vi "Select Dialog From Action.vi"(11 "Action":T2=enum."Terminal Properties") -> (3 "Dialog Selection":T1(ring))   [LabVIEW 2023]
uses:
  controls/action enum.ctl
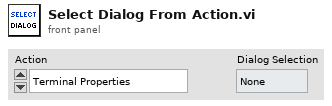
[diagram p1: front panel]
types:
  T1 = enum16{"None", "Cluster", "Property", "Method", "Class"}
  T2 = typedef "action enum.ctl" = enum16{"[NONE]", "Wire Bundle", "Wire Unbundle", "Terminal Unbundle", "Terminal Bundle", "Bundler Move Up", "Bundler Move Down", "Bundler Insert", "Bundler Remove", "Bundler Remove Unwired", "Bundler Rearrange", "In Place Insert", "In Place Remove", "In Place Remove Unwired", "In Place Rearrange", "Wire Properties", "Wire Method", "Terminal Properties", "Terminal Method", "Property Move Up", "Property Move Down", "Properties Insert", "Properties Remove", "Properties Remove Unwired", "Properties Rearrange", "Method Change", "Class for Constant", "Class For Control", "Class For Node", "Class Name to Clipboard"}
  T3 = cluster{"Action":T2, "Dialog Selection":enum16{"None", "Cluster", "Property", "Method", "Class"}}[]
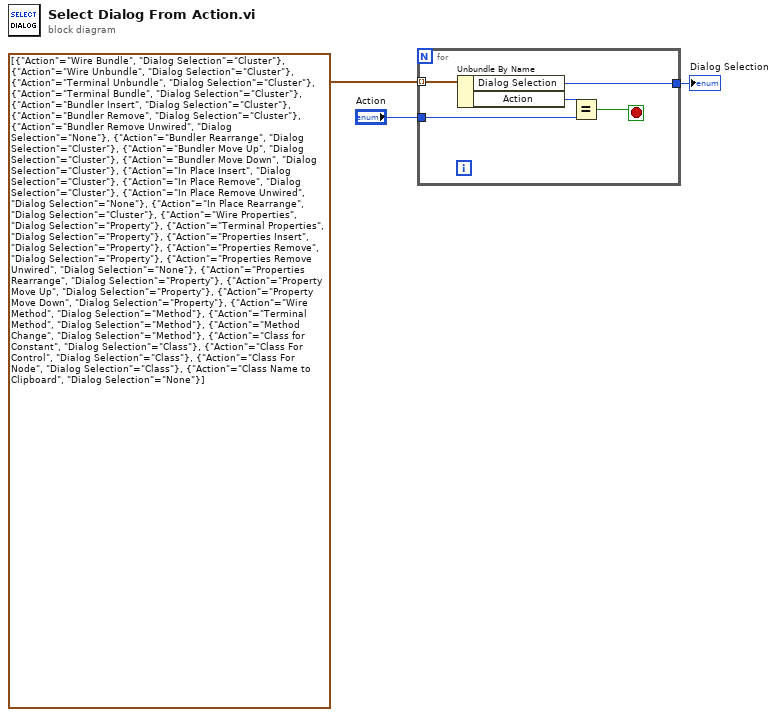
[diagram p0: block diagram]
diagram:
  n1 = for {
    tunnel: T3 [{"Action"=enum."Wire Bundle", "Dialog Selection"=enum."Cluster"}, {"Action"=enum."Wire Unbundle", "Dialog Selection"=enum."Cluster"}, {"Action"=enum."Terminal Unbundle", "Dialog Selection"=enum."Cluster"}, {"Action"=enum."Terminal Bundle", "Dialog Selection"=enum."Cluster"}, {"Action"=enum."Bundler Insert", "Dialog Selection"=enum."Cluster"}, {"Action"=enum."Bundler Remove", "Dialog Selection"=enum."Cluster"}, {"Action"=enum."Bundler Remove Unwired", "Dialog Selection"=enum."None"}, {"Action"=enum."Bundler Rearrange", "Dialog Selection"=enum."Cluster"}, {"Action"=enum."Bundler Move Up", "Dialog Selection"=enum."Cluster"}, {"Action"=enum."Bundler Move Down", "Dialog Selection"=enum."Cluster"}, {"Action"=enum."In Place Insert", "Dialog Selection"=enum."Cluster"}, {"Action"=enum."In Place Remove", "Dialog Selection"=enum."Cluster"}, {"Action"=enum."In Place Remove Unwired", "Dialog Selection"=enum."None"}, {"Action"=enum."In Place Rearrange", "Dialog Selection"=enum."Cluster"}, {"Action"=enum."Wire Properties", "Dialog Selection"=enum."Property"}, {"Action"=enum."Terminal Properties", "Dialog Selection"=enum."Property"}, {"Action"=enum."Properties Insert", "Dialog Selection"=enum."Property"}, {"Action"=enum."Properties Remove", "Dialog Selection"=enum."Property"}, {"Action"=enum."Properties Remove Unwired", "Dialog Selection"=enum."None"}, {"Action"=enum."Properties Rearrange", "Dialog Selection"=enum."Property"}, {"Action"=enum."Property Move Up", "Dialog Selection"=enum."Property"}, {"Action"=enum."Property Move Down", "Dialog Selection"=enum."Property"}, {"Action"=enum."Wire Method", "Dialog Selection"=enum."Method"}, {"Action"=enum."Terminal Method", "Dialog Selection"=enum."Method"}, {"Action"=enum."Method Change", "Dialog Selection"=enum."Method"}, {"Action"=enum."Class for Constant", "Dialog Selection"=enum."Class"}, {"Action"=enum."Class For Control", "Dialog Selection"=enum."Class"}, {"Action"=enum."Class For Node", "Dialog Selection"=enum."Class"}, {"Action"=enum."Class Name to Clipboard", "Dialog Selection"=enum."None"}] -> [w8] mode=indexing
    tunnel: "Action" -> [w6]
    tunnel: [w5] -> w2
    stop <- w4 stop-if-true
    n2 = Unbundle By Name(w8) -> ("Dialog Selection"=w5:T1, "Action"=w7:T2)
    n3 = Equal?(x=w7, y=w6) -> (x = y?=w4:bool)
  }
  "Dialog Selection" <- w2
